vi "MoveToPositionStr.vi"(11 "Position":string[](array[string])) -> ()   [LabVIEW 2020]
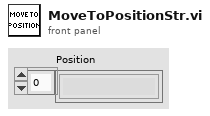
[diagram p1: front panel]
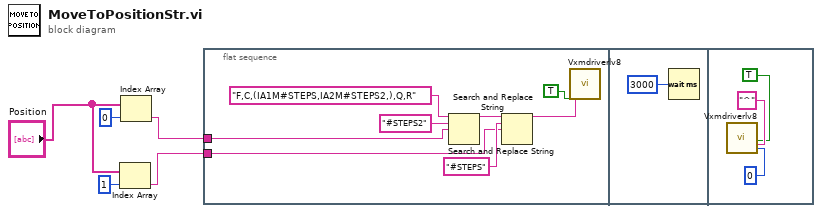
[diagram p0: block diagram]
diagram:
  n1 = Index Array(array="Position", index=1) -> (element=w1:string)
  n2 = Index Array(array="Position", index=0) -> (element=w2:string)
  n3 = flat-sequence {
    tunnel: w2 -> [w7]
    tunnel: w1 -> [w6]
    frame #0 {
      n4 = Search and Replace String(input string="F,C,(IA1M#STEPS,IA2M#STEPS2,),Q,R" ("Chars to send"), search string="#STEPS2", replace string=w7) -> (result string=w10:string)  [unwired: 5 in, 3 out]
      n5 = Search and Replace String(input string=w10, search string="#STEPS", replace string=w6) -> (result string=w11:string)  [unwired: 5 in, 3 out]
      n6 = call "Vxmdriverlv8.Vi"("Send\nchars\nto port"=TRUE, "Chars to send"=w11) -> ()  [unwired: 20 in, 6 out]
    }
    frame #1 {
      n7 = Wait (ms)(milliseconds to wait=u32 3000) -> ()  [unwired: 1 out]
    }
    frame #2 {
      n8 = call "Vxmdriverlv8.Vi"("Wait\nfor \nchar"=TRUE, "Char(s) to wait for"="^", "Char\nTimeout\nTime (ms)"=0) -> ()  [unwired: 19 in, 6 out]
    }
  }
